vi "SENS_CORR_COLL_GUID_DESC.vi"(0 "VISA IN":refnum<visa-resource-name>, 1 "Index":i32, 5 "error in":errorcluster, 7 "Channel":i32=1) -> (14 "VISA Out":refnum<visa-resource-name>, 18 "Description":string, 19 "error out":errorcluster)   [LabVIEW 2018, in "PNA-X.lvlib"]
doc: "SENSe:CORRection:COLLect:GUIDed:STEPs?\n(Read-only) Returns the number of measurement steps required to complete the current guided calibration. This command is sent after the SENS:CORR:COLL:GUID:INIT, SENS:CORR:COLL:GUID:CONN:PORT and SENS:CORR:COLL:GUID:CKIT:PORT commands.\n \nExamples\n SENS:CORR:COLL:GUID:STEP?\nsense2:correction:collect:guided:steps?\n \nReturn Type\n Numeric\n \nDefault\n Not Applicable"
uses:
  PNA-X.lvlib
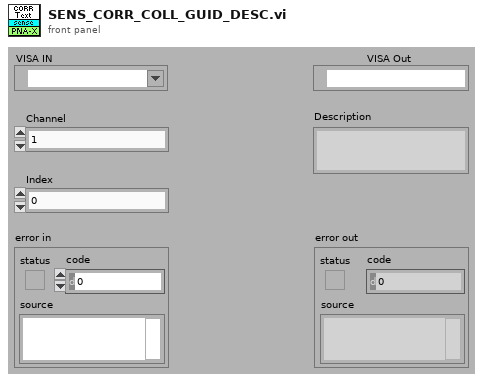
[diagram p1: front panel]
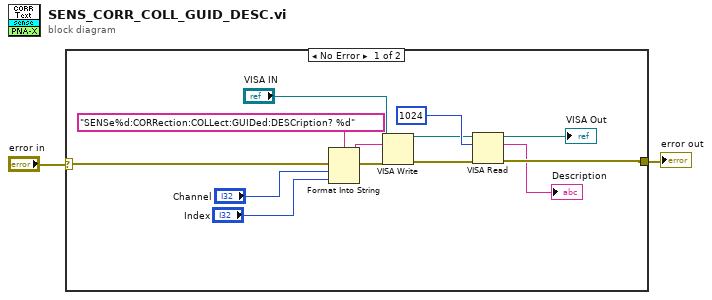
[diagram p0: block diagram]
diagram:
  n1 = case shown="No Error" "error in" {
    selector: "error in" -> [w15 w16]
    tunnel: [w6 w16] -> w1
    frame No Error {
      n2 = Format Into String(format string="SENSe%d:CORRection:COLLect:GUIDed:DESCription? %d" ("Cmdline"), error in=w15, "Channel", "Index") -> (resulting string=w13:string, error out=w14:errorcluster)  [unwired: 1 in]
      n3 = VISA Write(VISA resource name="VISA IN", write buffer=w13, error in (no error)=w14) -> (VISA resource name out=w8:refnum<visa-resource-name>, error out=w10:errorcluster)  [unwired: 1 out]
      n4 = VISA Read(VISA resource name=w8, byte count=1024, error in (no error)=w10) -> (VISA resource name out=→"VISA Out":refnum<visa-resource-name>, read buffer=→"Description":string, error out=w6:errorcluster)  [unwired: 1 out]
    }
    frame Error {
    }
  }
  "error out" <- w1
